vi "libssh2_knownhost_del.vi"(8 "error in (no error)":errorcluster, 10 "host key":T1, 11 "host key database":T2) -> (0 "error out":errorcluster)   [LabVIEW 2013, in "libssh2.lvlib"]
doc: "Delete a host key from from a host key database."
uses:
  libssh2.lvlib
  Host Key Database Refnum.ctl
  Host Key Refnum.ctl
  Not A Host Key Database.vi
  <vilib>/Utility/error.llb/Error Cluster From Error Code.vi
  Not A Host Key.vi
  Global Settings.vi
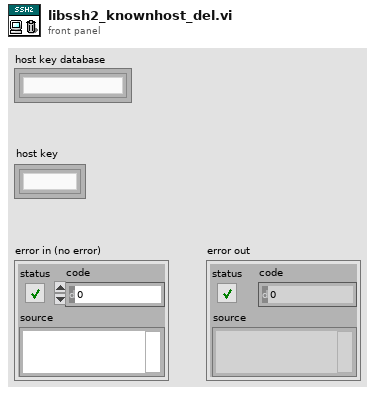
[diagram p1: front panel]
types:
  T1 = typedef "libssh2.lvlib/Host Key Refnum.ctl" = refnum<k1>
  T2 = typedef "libssh2.lvlib/Host Key Database Refnum.ctl" = refnum<k1>
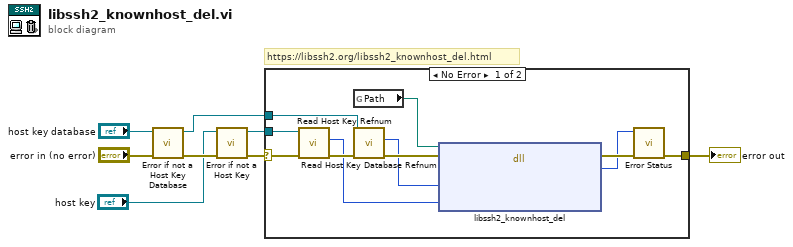
[diagram p0: block diagram]
diagram:
  # "https://libssh2.org/libssh2_knownhost_del.html"
  n1 = call "Error if not a Host Key Database.vi"("error in (no error)"="error in (no error)", "host key database"="host key database") -> ("error out"=w6:errorcluster, "host key database out"=w4:T2)  [unwired: 8 in]
  n2 = call "Error if not a Host Key.vi"("error in (no error)"=w6, "host key"="host key") -> ("error out"=w3:errorcluster, "host key out"=w1:T1)  [unwired: 8 in]
  n3 = case shown="No Error" w3 {
    selector: w3 -> [w19 w20]
    tunnel: [w18 w20] -> w8
    tunnel: w4 -> [w17 _]
    tunnel: w1 -> [w9 _]
    frame No Error {
      n4 = call "Read Host Key Refnum.vi"("error in (no error)"=w19, "host key"=w9) -> ("error out"=w11:errorcluster, "libssh2_knownhost*"=w10:u64)  [unwired: 8 in]
      n5 = global read "Global Settings.vi" "Path"() -> (w13:path)
      n6 = call "Read Host Key Database Refnum.vi"("error in (no error)"=w11, "host key database"=w17) -> ("error out"=w15:errorcluster, "LIBSSH2_KNOWNHOSTS*"=w14:u64)  [unwired: 8 in]
      n7 = dll-call lib="?" fn="libssh2_knownhost_del"(path in=w13, error in=w15, "hosts"=w14, "entry"=w10) -> (error out=w16:errorcluster, "return value"=w12:i32)  [unwired: 3 in, 1 out]
      n8 = call "Error Status.vi"("error in (no error)"=w16, "return value"=w12) -> ("error out"=w18:errorcluster)  [unwired: 8 in, 1 out]
    }
    frame Error {
    }
  }
  "error out" <- w8
